vi "FreqStep-Get Tone Amplitude.vi"(8 "error in (no error)":errorcluster, 9 "Level":T1, 11 "Inst Freq (Hz)":dbl[](array[numeric])) -> (0 "error out":errorcluster, 3 "Multiplier":dbl[](array[numeric]))   [LabVIEW 2015]
doc: "Interpolates calibration on instantaneous tone frequency to achieve constant power during a frequency transition."
uses:
  Controls/Level XCtl/Level Data.ctl
  Controls/Level XCtl/Level Units.ctl
  PXI DAQ VIs/DAQ Engine VIs/PXI Globals.vi
  Utility VIs/Math VIs/Linear to dB (scalar).vi
  Utility VIs/Math VIs/dB to Linear (1D).vi
  Controls/Level XCtl/Level XCtl.xctl
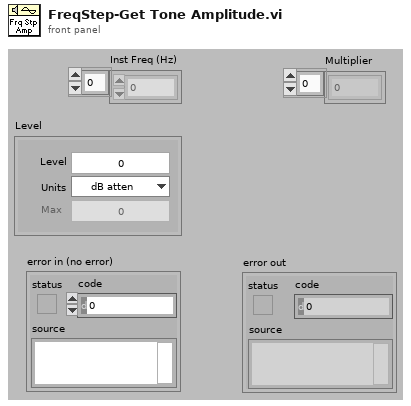
[diagram p1: front panel]
types:
  T1 = typedef "Level XCtl.xctl/Level Data.ctl" = cluster{"Level":dbl, "Units":T2, "Max":dbl, "Multiplier":dbl, "Cal File":path, "Cal":cluster{"Freq (Hz)":dbl[], "Mag (dB SPL)":dbl[], "Phase (deg)":dbl[]}}
  T2 = typedef "Level Units.ctl" = enum16{"dB atten", "dB SPL", "dB re 1 Vrms", "dB V/Hz½", "mW", "dB SL"}
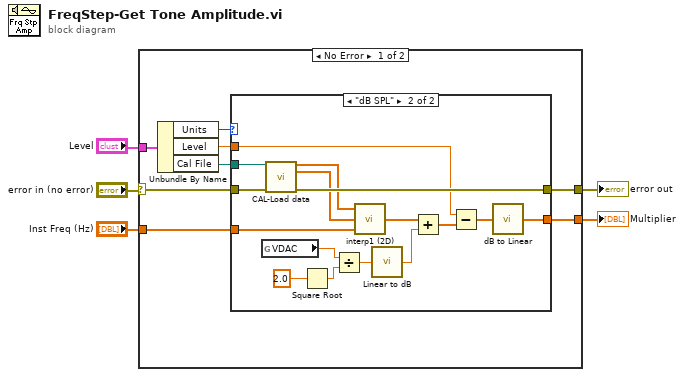
[diagram p0: block diagram]
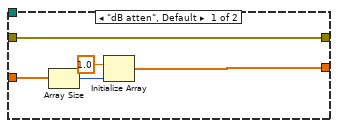
[diagram p2: hidden frame]
diagram:
  n1 = case shown="No Error" "error in (no error)" {
    selector: "error in (no error)" -> [w8 w35]
    tunnel: "Level" -> [w13 _]
    tunnel: "Inst Freq (Hz)" -> [w11 _]
    tunnel: [w10 _] -> w2
    tunnel: [w7 w35] -> w1
    frame No Error {
      n2 = Unbundle By Name(w13) -> ("Units"=w12:T2, "Level"=w6:dbl, "Cal File"=w9:path)
      n3 = case shown="\"dB SPL\"" w12 {
        tunnel: w11 -> [w18 w29]
        tunnel: [w15 w20] -> w10
        tunnel: w9 -> [_ w34]
        tunnel: w8 -> [w14 w33]
        tunnel: [w14 w32] -> w7
        tunnel: w6 -> [_ w22]
        frame "dB atten", Default {
          n4 = Array Size(array=w18) -> (size(s)=w17:i32)
          n5 = Initialize Array(1.0 ("element"), w17) -> (w15:dbl[])
        }
        frame "dB SPL" {
          n6 = global read "PXI Globals.vi" "VDAC"() -> (w19:dbl)
          n7 = call "CAL-Load data.vi"("user path"=w34, "error in (no error)"=w33) -> ("Frequency (Hz)"=w31:dbl[], "Mag"=w30:dbl[], "error out"=w32:errorcluster)  [unwired: 6 in, 5 out]
          n8 = Square Root(x=2.0) -> (sqrt(x)=w28:dbl)
          n9 = Divide(x=w19, y=w28) -> (x/y=w26:dbl)
          n10 = call "interp1 (2D).vi"("U"=w29, "Y"=w30, "X"=w31) -> ("V"=w25:dbl[])
          n11 = call-poly "Linear to dB.vi"("Linear"=w26) -> ("dB"=w24:dbl)
          n12 = Add(x=w25, y=w24) -> (x+y=w23:dbl[])
          n13 = Subtract(x=w22, y=w23) -> (x-y=w21:dbl[])
          n14 = call-poly "dB to Linear.vi"("dB"=w21) -> ("linear"=w20:dbl[])
        }
      }
    }
    frame Error {
    }
  }
  "error out" <- w1
  "Multiplier" <- w2
